vi "Initialize and Register Tasks.vi"(8 "error in":errorcluster, 11 "sequence context in":refnum<k7>) -> (0 "error out":errorcluster)   [LabVIEW 2021, in "NIDAQmxMeasurement.lvlib"]
doc: "This VI will get called as part of the TestStand ProcessSetup sequence. It creates and registers all DAQmx tasks in the Session Mangement Service."
uses:
  NIDAQmxMeasurement.lvlib
  <vilib>/gRPC/Generated APIs/ni/measurementlink/sessionmanagement/v1/RPC Messages/ni_measurementlink_PinMapContext.ctl
  <vilib>/Plug-In SDKs/Clients/Session Management V1/Session Reservation/Initialize and Close Session Behavior.ctl
  <vilib>/Plug-In SDKs/TestStand/NI Pin Map TestStand.lvlib
  <vilib>/Plug-In SDKs/Clients/Session Management V1/Session Reservation/Session Reservation.lvclass
  Source/Sessions/niDAQmx/Session Management niDAQmx.lvlib
  <vilib>/gRPC/Generated APIs/ni/measurementlink/sessionmanagement/v1/ni.measurementlink.sessionmanagement.v1.api.lvlib
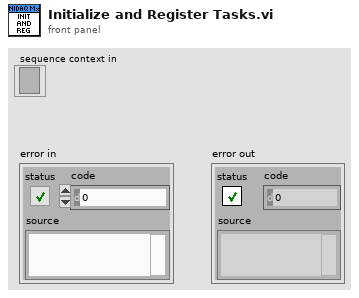
[diagram p1: front panel]
types:
  T1 = typedef "NI Session Management V1 Client.lvlib/Session Reservation.lvclass/Initialize and Close Session Behavior.ctl" = enum16{"Auto", "Initialize and Close", "Attach and Detach", "Initialize and Detach", "Attach and Close"}
  T2 = typedef "ni.measurementlink.sessionmanagement.v1.api.lvlib/ni_measurementlink_PinMapContext.ctl" = cluster{"pin_map_id":string, "sites":i32[]}
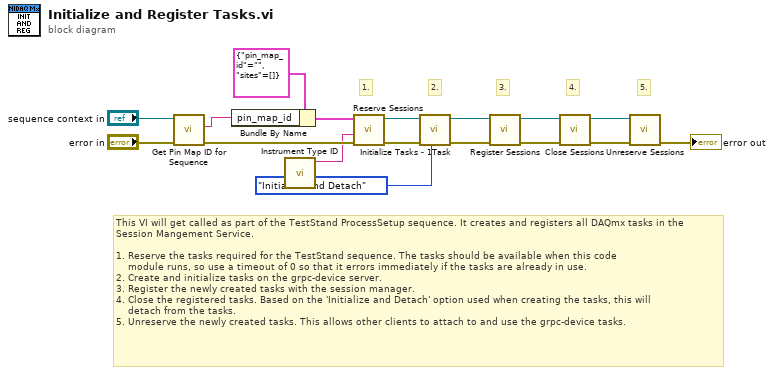
[diagram p0: block diagram]
diagram:
  # "4."
  # "5."
  # "3."
  # "2."
  # "1."
  # "This VI will get called as part of the TestStand ProcessSetup sequence. It creates and registers all DAQmx tasks in the\nSession Mangement Service.\n\n1. Reserve the tasks required for the TestStand sequence. The tasks should be available when this code\n    module runs, so use a timeout of 0 so that it errors immediately if the tasks are already in use.  \n2. Create and initialize tasks on the grpc-device server.\n3. Register the newly created tasks with the session manager.\n4. Close the registered tasks. Based on the 'Initialize and Detach' option used when creating the tasks, this will\n    detach from the tasks.\n5. Unreserve the newly created tasks. This allows other clients to attach to and use the grpc-device tasks."
  n1 = call <vilib>:"Get Pin Map ID for Sequence.vi"("error in"="error in", "sequence context in"="sequence context in") -> ("error out"=w12:errorcluster, "pin map id"=w14:string)  [unwired: 7 in, 1 out]
  n2 = Bundle By Name(cluster=T2 {"pin_map_id"="", "sites"=[]} ("pin map context"), "pin_map_id"=w14) -> (w13:T2)
  n3 = call "Instrument Type ID.vi"() -> ("instrument type id"=w11:string)  [unwired: 11 in]
  n4 = call <vilib>:"Reserve Sessions.vi"("error in"=w12, "instrument type id"=w11, "pin map context"=w13) -> ("error out"=w6:errorcluster, "session reservation out"=w10:refnum<class "Session Reservation.lvclass">)  [unwired: 7 in]
  n5 = call "Initialize Tasks - 1Task.vi"("initialize and close session behavior"=Initialize_and_Close_Session_Behavior."Initialize and Detach", "error in"=w6, "session reservation in"=w10) -> ("error out"=w5:errorcluster, "session reservation out"=w9:refnum<class "Session Reservation.lvclass">)  [unwired: 5 in, 2 out]
  n6 = call <vilib>:"Register Sessions.vi"("error in"=w5, "session reservation in"=w9) -> ("error out"=w4:errorcluster, "session reservation out"=w8:refnum<class "Session Reservation.lvclass">)  [unwired: 8 in]
  n7 = call <vilib>:"Close Sessions.vi"("error in"=w4, "session reservation in"=w8) -> ("error out"=w3:errorcluster, "session reservation out"=w7:refnum<class "Session Reservation.lvclass">)  [unwired: 8 in]
  n8 = call <vilib>:"Unreserve Sessions.vi"("error in"=w3, "session reservation in"=w7) -> ("error out"=→"error out":errorcluster)  [unwired: 9 in]
